vi "Graph Attributes Initialize.vi"(10 "Graph Ref":refnum<vi>, 11 "Graph to initialize Refs":refnum<vi>[](array[refnum])) -> ()   [LabVIEW 2023]
doc: "Use this VI to initialize graph attributes such as Plot Color, Point Color, and Cursor Color based on the reference graph."
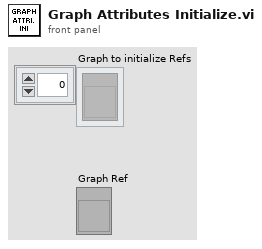
[diagram p1: front panel]
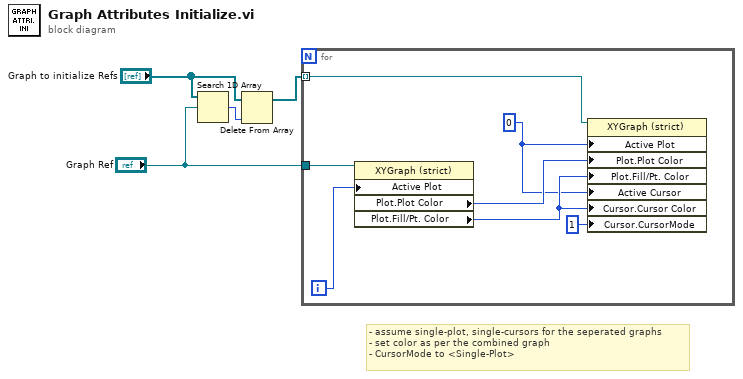
[diagram p0: block diagram]
diagram:
  # "- assume single-plot, single-cursors for the seperated graphs\n- set color as per the combined graph\n- CursorMode to <Single-Plot>"
  n1 = Search 1D Array(1D array="Graph to initialize Refs", element="Graph Ref") -> (index of element=w2:i32)  [unwired: 1 in]
  n2 = Delete From Array(array="Graph to initialize Refs", index=w2) -> (array with subset deleted=w1:refnum<vi>[])  [unwired: 1 in, 1 out]
  n3 = for {
    tunnel: "Graph Ref" -> [w11]
    tunnel: w1 -> [w6] mode=indexing
    i -> [w8]
    w7 = u32 0 ("Active Plot")
    n4 = property class="XYGraph (strict)"(reference=w11, "Active Plot"=w8) -> ("Plot.Plot Color"=w10:u32, "Plot.Fill/Pt. Color"=w9:u32)  [unwired: 1 in, 2 out]
    n5 = property class="XYGraph (strict)"(reference=w6, "Active Plot"=w7, "Plot.Plot Color"=w10, "Plot.Fill/Pt. Color"=w9, "Active Cursor"=w7, "Cursor.Cursor Color"=w9, "Cursor.CursorMode"=u32 1 ("Cursor.Cursor Mode")) -> ()  [unwired: 1 in, 2 out]
  }
